vi "Update UI.vi"(0 "DAQ Controller in":refnum<class "QPDController.lvclass">, 5 "DataExchange":T2, 11 "error in (no error)":errorcluster) -> (4 "DAQ Controller out":refnum<class "QPDController.lvclass">, 15 "error out":errorcluster)   [LabVIEW 2020]
uses:
  QPDController.lvclass
  E:/Development/DevHardSoftware/MicroscopyFramework/Model/Hardware Abstraction Layer/Component/GenericActor/GenericActor/GenericController.lvclass
  C:/Program Files/National Instruments/LabVIEW 2020/vi.lib/ActorFramework/Actor/Actor.lvclass
  E:/Development/DevHardSoftware/MicroscopyFramework/Interface/DataGenerator/DataGenerator.lvclass
  E:/Development/DevHardSoftware/MicroscopyFramework/Interface/DataListener/DataListener.lvclass
  E:/Development/DevHardSoftware/MicroscopyFramework/Interface/ErrorHandler/ErrorHandler.lvclass
  E:/Development/DevHardSoftware/MicroscopyFramework/ViewController/QPDController/QPDController.lvclass
  Model/Hardware Abstraction Layer/Component/Device/Device/DataExchange.ctl
  Interface/DataListener/DataListener.lvclass
panel:
  in  "Cluster":T1 {"QPD  Sum" format="%#_13g"; "QPD Voltage Y" format="%#_13g"; "QPD Voltage X" format="%#_13g"}
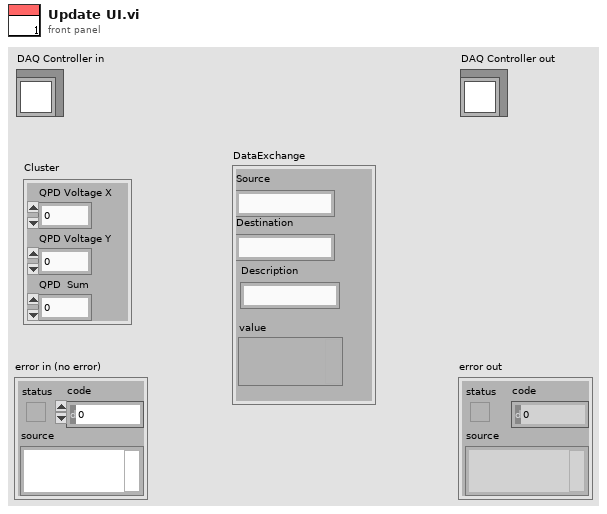
[diagram p1: front panel]
types:
  T1 = cluster{"QPD Voltage X":dbl, "QPD Voltage Y":dbl, "QPD  Sum":dbl}
  T2 = typedef "DataListener.lvclass/DataExchange.ctl" = cluster{"Source":string, "Destination":string, "Description":string, "value":variant}
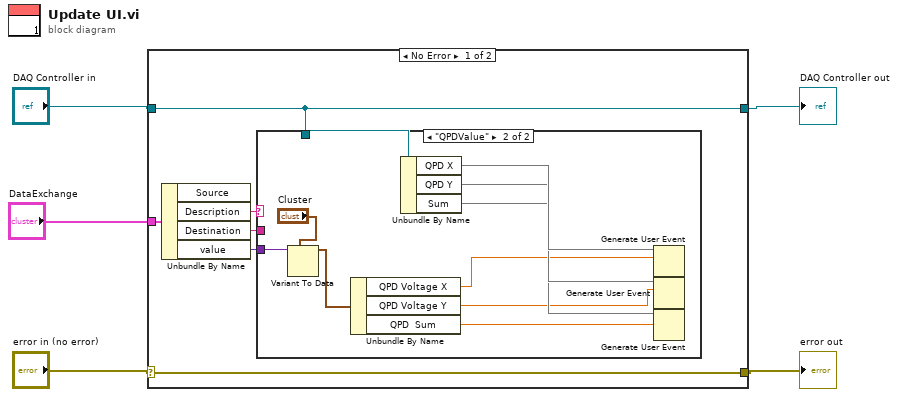
[diagram p0: block diagram]
diagram:
  n1 = case shown="No Error" "error in (no error)" {
    selector: "error in (no error)" -> [w11 w23]
    tunnel: [w11 w23] -> w2
    tunnel: [w6 w22] -> w3
    tunnel: "DAQ Controller in" -> [w6 w22]
    tunnel: "DataExchange" -> [w10 _]
    frame No Error {
      n2 = Unbundle By Name(w10) -> ("Description"=w7:string, "Destination"=w8:string, "value"=w9:variant)  [unwired: 1 out]
      n3 = case shown="\"QPDValue\"" w7 {
        tunnel: w9 -> [_ w21]
        tunnel: w8 -> [_ _]
        tunnel: w6 -> [_ w20]
        frame "False", Default {
        }
        frame "QPDValue" {
          n4 = Variant To Data(type="Cluster", Variant=w21) -> (data=w16:T1)  [unwired: 1 in, 1 out]
          n5 = Unbundle By Name(w16) -> ("QPD Voltage X"=w15:dbl, "QPD Voltage Y"=w14:dbl, "QPD  Sum"=w13:dbl)
          n6 = Unbundle By Name(w20) -> ("QPD X"=w19, "QPD Y"=w18, "Sum"=w17)
          n7 = Generate User Event(user event=w19, event data cluster=w15) -> ()  [unwired: 2 in, 2 out]
          n8 = Generate User Event(user event=w18, event data cluster=w14) -> ()  [unwired: 2 in, 2 out]
          n9 = Generate User Event(user event=w17, event data cluster=w13) -> ()  [unwired: 2 in, 2 out]
        }
      }
    }
    frame Error {
    }
  }
  "error out" <- w2
  "DAQ Controller out" <- w3
